vi "Subtract Partial Waveform.vi"(3 "Offset (0)":i32, 4 "Subsignal":waveform(dbl)[](array[waveform]), 5 "Signal":waveform(dbl)[](array[waveform])) -> (1 "Difference":waveform(dbl)[](array[waveform]))   [LabVIEW 2013]
panel:
  out "Index Difference":i32
  out "Waveform Graph 4":waveform(dbl)[](graph)
  out "Waveform Graph 3":waveform(dbl)[](graph)
  out "Waveform Graph 2":waveform(dbl)[](graph)
  out "Waveform Graph":waveform(dbl)[](graph)
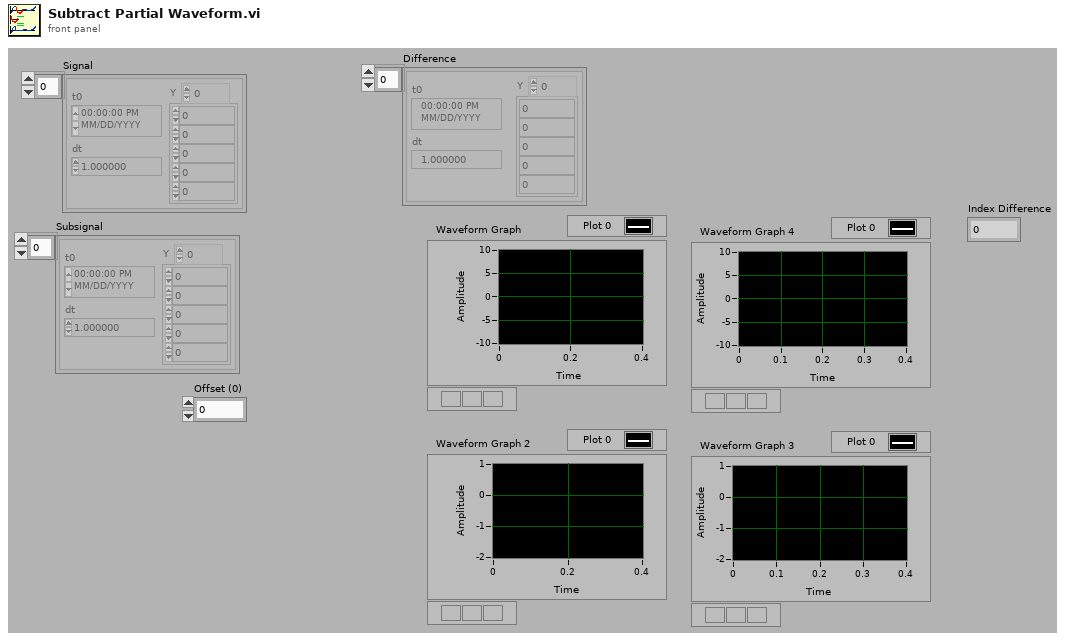
[diagram p1: front panel]
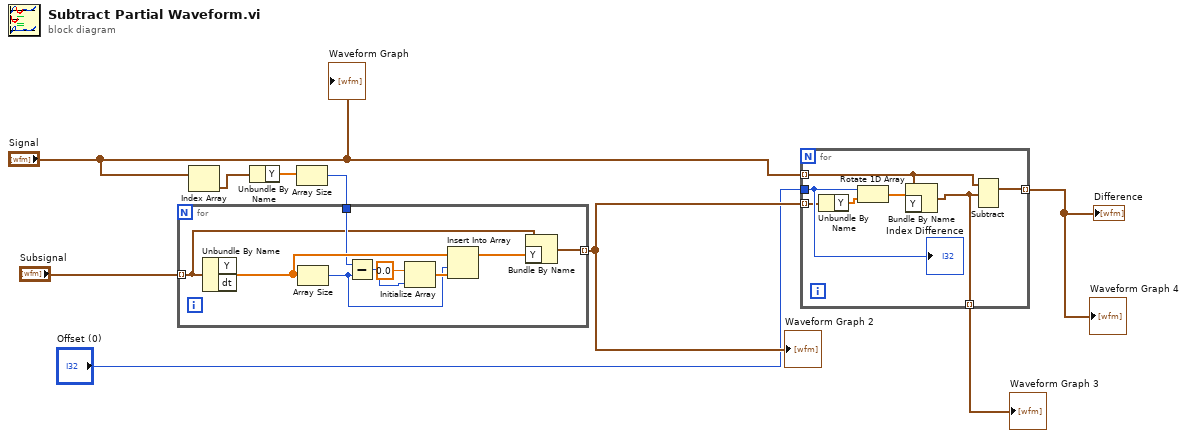
[diagram p0: block diagram]
diagram:
  n1 = Index Array(array="Signal") -> (element=w3:waveform(dbl))  [unwired: 1 in]
  n2 = Unbundle By Name(w3) -> ("Y"=w5:dbl[])
  n3 = Array Size(array=w5) -> (size(s)=w2:i32)
  n4 = for {
    tunnel: [w10] -> w7 mode=indexing
    tunnel: "Subsignal" -> [w11] mode=indexing
    tunnel: w2 -> [w13]
    n5 = Unbundle By Name(w11) -> ("Y"=w14:dbl[])  [unwired: 1 out]
    n6 = Array Size(array=w14) -> (size(s)=w15:i32)
    n7 = Subtract(x=w13, y=w15) -> (x-y=w17:i32)
    n8 = Initialize Array(0.0 ("element"), w17) -> (w18:dbl[])
    n9 = Insert Into Array(array=w14, index=w15, new element=w18) -> (w12:dbl[])
    n10 = Bundle By Name(cluster=w11, "Y"=w12) -> (w10:waveform(dbl))
  }
  "Waveform Graph 2" <- w7
  n11 = for {
    tunnel: [w19] -> w9 mode=indexing
    tunnel: w7 -> [w23] mode=indexing
    tunnel: [w25] -> w8 mode=indexing
    tunnel: "Signal" -> [w20] mode=indexing
    tunnel: "Offset (0)" -> [w24]
    n12 = Unbundle By Name(w23) -> ("Y"=w22:dbl[])
    n13 = Rotate 1D Array(1:w22, 2:w24) -> (0:w21:dbl[])
    n14 = Bundle By Name(cluster=w20, "Y"=w21) -> (w19:waveform(dbl))
    n15 = Subtract(1:w19, 2:w20) -> (0:w25:waveform(dbl))  [unwired: 1 in, 1 out]
    "Index Difference" <- w24
  }
  "Waveform Graph 3" <- w9
  "Waveform Graph 4" <- w8
  "Difference" <- w8
  "Waveform Graph" <- "Signal"
